vi "Set Interface.vi"(10 "Interface":refnum<class "Plugin Interface.lvclass">, 11 "Transceiver Thread in":refnum<class "Plugin Thread.lvclass">) -> (3 "Transceiver Thread out":refnum<class "Plugin Thread.lvclass">)   [LabVIEW 2017, in "DSF Core.lvlib" / "Plugin Thread.lvclass"]
uses:
  Plugin Thread.lvclass
  Interfaces/Transceiver Interface/Plugin Interface.lvclass
  Plugin Thread.lvclass/Plugin Thread.ctl
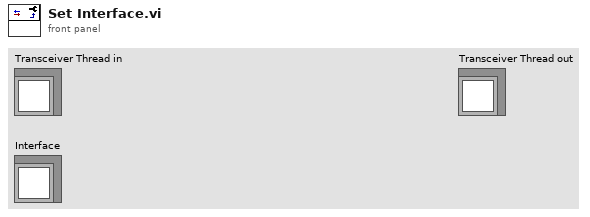
[diagram p1: front panel]
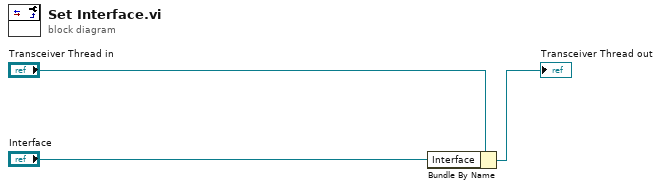
[diagram p0: block diagram]
diagram:
  n1 = Bundle By Name(cluster="Transceiver Thread in", "Interface"="Interface") -> (→"Transceiver Thread out":refnum<class "Plugin Thread.lvclass">)
